vi "PROCESS_CTRL_VI.vi"(7 "simulazione":bool, 8 "error in (no error)":errorcluster, 10 "SINOTTICO NM":refnum<vi>, 11 "Queue Name":string) -> (0 "error out":errorcluster, 2 "Stopped":bool)   [LabVIEW 2016]
uses:
  TypeDef/Cluster MISURE.ctl
  TypeDef/MISURE NM.ctl
  TypeDef/Cluster misure ALL.ctl
  TypeDef/Cluster NI.ctl
  cDAQ_PLC Folder/controls/StatoAO_cdaq.ctl
  cDAQ_PLC Folder/controls/statoDO_Cdaq.ctl
  TypeDef/MISURE WT.ctl
  TypeDef/ClusterRes.ctl
  TypeDef/INTERFACCIA.ctl
  TypeDef/Lista AO sistema.ctl
  TypeDef/DOinterfaccia.ctl
  cDAQ_PLC Folder/ST1200_LIST_IO/STATO PLC 1.ctl
  cDAQ_PLC Folder/ST1200_LIST_IO/Uscite PLC 1.ctl
  cDAQ_PLC Folder/controls/statoAO_plc_1.ctl
  cDAQ_PLC Folder/ST1200_LIST_IO/StatoDO_PLC_1.ctl
  SINUS PENTA SANTERNO/controls/Parametri inverter letti.ctl
  TypeDef/SINOTTICO NM.ctl
  Globals.vi
panel:
  out "Setup pressione":dbl[](array[numeric])
  out "CTRL BV 3":cluster{"ON":bool, "OFF":bool}
  out "CTRL BV 2":cluster{"ON":bool, "OFF":bool}
  out "Stato Soglie":bool[](array[boolean])
  out "Pressione misurata":dbl
  out "Set Pressione":dbl
  out "Controllo Pressione":bool
  out "# in queue":i32
  out "STATO":string
  out "LOOP TIME (ms)":u32
  # "OK"
  # "BELOW RANGE"
  # "OVER RANGE"
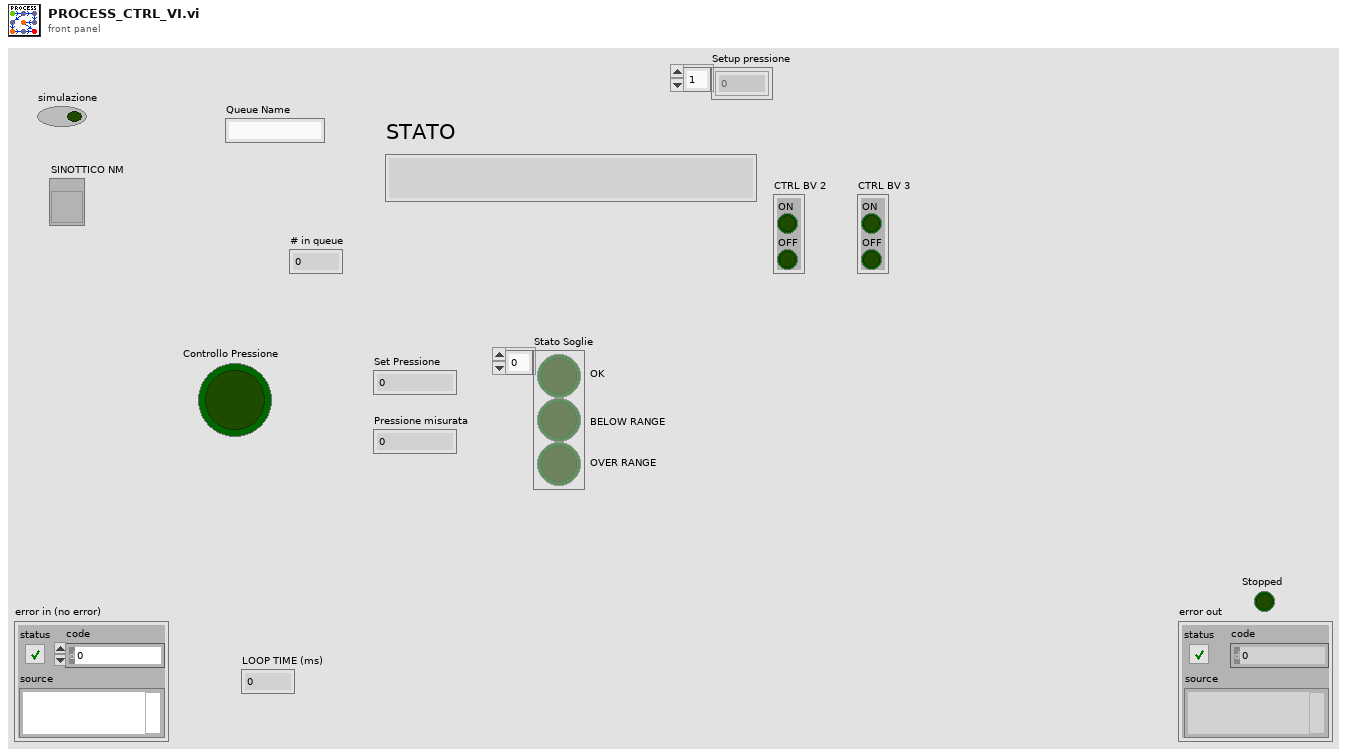
[diagram p1: front panel]
types:
  T1 = typedef "SINOTTICO NM.ctl" = cluster{"BooleanV 1":bool, "BooleanV 2":bool, "BooleanV 3":bool, "BooleanV 4":bool, "BooleanV 5":bool, "BooleanV 6":bool, "CTRL BV 2":cluster{"ON":bool, "OFF":bool}, "CTRL BV 3":cluster{"ON":bool, "OFF":bool}, "CTRL BV 4":cluster{"ON":bool, "OFF":bool}, "CTRL BV 5":cluster{"ON":bool, "OFF":bool}, "CTRL BV 6":cluster{"ON":bool, "OFF":bool}, "MTR 1":bool, "DN40%":dbl, "DN100%":dbl, "DN250%":dbl, "DN32":dbl, "DN100":dbl, "DN250":dbl, "MTR 2":bool, "BooleanV 7":bool, "BooleanV 8":bool, "DN25%":dbl, "DN250_c":dbl, "CTRL BV 7":cluster{"ON":bool, "OFF":bool}, "CTRL BV 8":cluster{"ON":bool, "OFF":bool}, "DN300%":dbl, "H 2 [bar]":dbl, "H 1 [bar]":dbl, "Rpm\nTorsiometro":dbl, "Coppia\nTorsiometro":dbl, "Sonda Velocità":dbl, "T 2 [°C]":dbl, "T 1 [°C]":dbl, "P [bar]":dbl, "Livello [m]":dbl, "MTR 3":bool, "SEL DN40":bool, "SEL DN100":bool, "SEL DN250":bool, "SEL DN300":bool, "SEL DN25":bool}
  T2 = typedef "Cluster MISURE.ctl" = cluster{"MISURE NM":T3, "MISURE ALL":T4}
  T3 = typedef "MISURE NM.ctl" = cluster{"Banco":string, "Anno":string, "Numero":string, "Ntabella":string, "Misura":string, "Tipo Prova":string, "ProgressivoAcq":string, "Descrizione":string, "Data_ora":string, "t. acq [h:m:s]":string, "t. acq [min]":string, "t. acq [s]":string, "n [rpm]":string, "f [Hz]":string, "U1[V]":string, "U2 [V]":string, "U3 [V]":string, "U123_media [V]":string, "I1[A]":string, "I2[A]":string, "I3[A]":string, "I123_media [A]*I":string, "I_123_sbil [%]":string, "Ulin[V]":string, "Uc [V]":string, "Uaux [V]":string, "Ilin[A]*I":string, "Imar[A]":string, "Iaux[A]":string, "Uarm[V]":string, "Uecc[V]":string, "Iarm[A]*I":string, "Iecc[A]":string, "pf":string, "P1 [W]":string, "P1 [kW]":string, "P1arm[W]":string, "P1ecc[W]":string, "Parm[kW]":string, "P1ecc[kW]":string, "Cond[uF]":string, "P1_linea_6fili[W]":string, "P1_linea_6fili[kW]":string, "eta_gr_6fili [%]":string, "eta_inverter_6fili [%]":string, "pf_linea_6fili":string, "U4 [V]":string, "U5 [V]":string, "U6 [V]":string, "U456_media [V]":string, "I4 [A]":string, "I5 [A]":string, "I6 [A]":string, "I456_media [A]":string, "C [Nm]*C":string, "Cric [Nm]":string, "Cric\\Cnom":string, "Iric[A]":string, "Iric\\Inom":string, "P2_mecc [W]":string, "P2_mecc [kW]":string, "eta motore [%]":string, "Scorr[%]":string, "Tamb[°C]":string, "R1[ohm]":string, "R2[ohm]":string, "R3[ohm]":string, "DT_R1[°C]":string, "DT_R2[°C]":string, "DT_R3[°C]":string, "R_marcia[ohm]":string, "R_aux[ohm]":string, "DT_marcia[°C]":string, "DT_aux[°C]":string, "R_Arm[ohm]":string, "R_Ecc[ohm]":string, "DT_Arm[°C]":string, "DT_Ecc[°C]":string, "TambFreddo[°C]":string, "R1_freddo[ohm]":string, "R2_freddo[ohm]":string, "R3_freddo[ohm]":string, "R_Marcia_freddo[ohm]":string, "R_Aux_freddo[ohm]":string, "R_Arm_freddo[ohm]":string, "R_Ecc_freddo[ohm]":string, "Tc1":string, "Tc2":string, "Tc3":string, "Tc4":string, "Tc5":string, "Tc6":string, "Tc7":string, "Tc8":string, "Vibr 1":string, "Vibr 2":string, "Vibr 3":string, "Scorta 1":string, "Scorta 2":string, "Scorta 3":string, "Scorta 4":string, "Scorta 5":string, "Scorta 6":string, "Scorta 7":string, "Scorta 8":string, "Scorta 9":string, "Scorta 10":string}
  T4 = typedef "Cluster misure ALL.ctl" = cluster{"Cluster READ NI":T5, "MISURE WT":T8, "Resistenze Resistomat":T9, "INTERFACCIA":T10, "FREDDO resistomat":cluster{"Res Ch1":dbl, "Res Ch2":dbl, "tAMB":dbl, "Res Ch3":dbl}, "STATO PLC":T15, "Res Ch2":dbl, "Res Ch2 2":dbl, "FREDDO res meter":cluster{"Res Ch1":dbl, "Res Ch2":dbl, "tAMB":dbl, "Res Ch3":dbl}, "Resistenze Res Meter":T9, "READ SINUS PENTA":T19}
  T5 = typedef "Cluster NI.ctl" = cluster{"AI (0-10V)":cluster{"AI 0":dbl, "AI 1":dbl, "AI 2":dbl, "AI 3":dbl, "AI 4":dbl, "AI 5":dbl, "AI 6":dbl, "AI 7":dbl, "AI 8":dbl, "AI 9":dbl, "AI 10":dbl, "AI 11":dbl, "AI 12":dbl, "AI 13":dbl, "AI 14":dbl, "AI 15":dbl, "AI 16":dbl, "AI 17":dbl, "AI 18":dbl, "AI 19":dbl, "AI 20":dbl, "AI 21":dbl, "AI 22":dbl, "AI 23":dbl, "AI 24":dbl, "AI 25":dbl, "AI 26":dbl, "AI 27":dbl, "AI 28":dbl, "AI 29":dbl, "AI 30":dbl, "AI 31":dbl}, "StatoAO_Cdaq[0-10V]":cluster{"AO 1":dbl, "AO 2":dbl, "AO 3":dbl, "AO 4":dbl}, "Contatori [rpm]":cluster{"RPM 1":dbl, "RPM 2":dbl}, "StatoAO_Cdaq [4-20mA]":T6, "StatoDO_Cdaq":T7, "DI":cluster{"Scorta 0":bool, "Scorta 1":bool, "Scorta 2":bool, "Scorta 3":bool, "Scorta 4":bool, "Scorta 5":bool, "Scorta 6":bool, "Scorta 7":bool, "Scorta 8":bool, "Scorta 9":bool, "Scorta 10":bool, "Scorta 11":bool, "Scorta 12":bool, "Scorta 13":bool, "Scorta 14":bool, "Scorta 15":bool, "Scorta 16":bool, "Scorta 17":bool, "Scorta 18":bool, "Scorta 19":bool, "Scorta 20":bool, "Scorta 21":bool, "Scorta 22":bool, "Scorta 23":bool, "Scorta 24":bool, "Scorta 25":bool, "Scorta 26":bool, "Scorta 27":bool, "Scorta 28":bool, "Scorta 29":bool, "Scorta 30":bool, "Scorta 31":bool}, "AI (4-20mA)":cluster{"AI 0":dbl, "AI 1":dbl, "AI 2":dbl, "AI 3":dbl, "AI 4":dbl, "AI 5":dbl, "AI 6":dbl, "AI 7":dbl, "AI 8":dbl, "AI 9":dbl, "AI 10":dbl, "AI 11":dbl, "AI 12":dbl, "AI 13":dbl, "AI 14":dbl, "AI 15":dbl}}
  T6 = typedef "StatoAO_cdaq.ctl" = cluster{"Cdaq_AO [0-10V] 0":dbl, "Cdaq_AO [0-10V] 1":dbl, "Cdaq_AO [0-10V] 2":dbl, "Cdaq_AO [0-10V] 3":dbl, "Cdaq_AO [4-20mA] 0":dbl, "Cdaq_AO [4-20mA] 1":dbl, "Cdaq_AO [4-20mA] 2":dbl, "Cdaq_AO [4-20mA] 3":dbl, "Cdaq_AO [4-20mA] 4":dbl, "Cdaq_AO [4-20mA] 5":dbl, "Cdaq_AO [4-20mA] 6":dbl, "Cdaq_AO [4-20mA] 7":dbl}
  T7 = typedef "statoDO_Cdaq.ctl" = cluster{"Scorta 0":bool, "Scorta 1":bool, "Scorta 2":bool, "Scorta 3":bool, "Scorta 4":bool, "Scorta 5":bool, "Scorta 6":bool, "Scorta 7":bool, "Scorta 8":bool, "Scorta 9":bool, "Scorta 10":bool, "Scorta 11":bool, "Scorta 12":bool, "Scorta 13":bool, "Scorta 14":bool, "Scorta 15":bool, "Scorta 16":bool, "Scorta 17":bool, "Scorta 18":bool, "Scorta 19":bool, "Scorta 20":bool, "Scorta 21":bool, "Scorta 22":bool, "Scorta 23":bool, "Scorta 24":bool, "Scorta 25":bool, "Scorta 26":bool, "Scorta 27":bool, "Scorta 28":bool, "Scorta 29":bool, "Scorta 30":bool, "Scorta 31":bool}
  T8 = typedef "MISURE WT.ctl" = cluster{"URMS 1":dbl, "IRMS 1":dbl, "P 1":dbl, "S 1":dbl, "Q 1":dbl, "LAMBDA 1":dbl, "PHI 1":dbl, "F U 1":dbl, "F I 1":dbl, "NONE 1":dbl, "URMS 2":dbl, "IRMS 2":dbl, "P 2":dbl, "S 2":dbl, "Q 2":dbl, "LAMBDA 2":dbl, "PHI 2":dbl, "F U 2":dbl, "F I 2":dbl, "NONE 2":dbl, "URMS 3":dbl, "IRMS 3":dbl, "P 3":dbl, "S 3":dbl, "Q 3":dbl, "LAMBDA 3":dbl, "PHI 3":dbl, "F U 3":dbl, "F I 3":dbl, "NONE 3":dbl, "URMS 4":dbl, "IRMS 4":dbl, "P 4":dbl, "S 4":dbl, "Q 4":dbl, "LAMBDA 4":dbl, "PHI 4":dbl, "F U 4":dbl, "F I 4":dbl, "NONE 4":dbl, "URMS 5":dbl, "IRMS 5":dbl, "P 5":dbl, "S 5":dbl, "Q 5":dbl, "LAMBDA 5":dbl, "PHI 5":dbl, "F U 5":dbl, "F I 5":dbl, "NONE 5":dbl, "URMS 6":dbl, "IRMS 6":dbl, "P 6":dbl, "S 6":dbl, "Q 6":dbl, "LAMBDA 6":dbl, "PHI 6":dbl, "F U 6":dbl, "F I 6":dbl, "NONE 6":dbl, "URMS SIGMA":dbl, "IRMS SIGMA":dbl, "P SIGMA":dbl, "S SIGMA":dbl, "Q SIGMA":dbl, "LAMBDA SIGMA":dbl, "PHI SIGMA":dbl, "F U SIGMA":dbl, "F I SIGMA":dbl, "NONE 7":dbl, "URMS SIGMB":dbl, "IRMS SIGMB":dbl, "P SIGMB":dbl, "S SIGMB":dbl, "Q SIGMB":dbl, "LAMBDA SIGMB":dbl, "PHI SIGMB":dbl, "F U SIGMB":dbl, "F I SIGMB":dbl, "NONE 8":dbl, "URMS SIGMC":dbl, "IRMS SIGMC":dbl, "P SIGMC":dbl, "S SIGMC":dbl, "Q SIGMC":dbl, "LAMBDA SIGMC":dbl, "PHI SIGMC":dbl, "F U SIGMC":dbl, "F I SIGMC":dbl, "NONE 9":dbl}
  T9 = typedef "ClusterRes.ctl" = cluster{"Res Ch1":dbl, "Res Ch2":dbl, "Res Ch3":dbl}
  T10 = typedef "INTERFACCIA.ctl" = cluster{"AI":cluster{"Portate":T11[], "Pressioni":T11[], "Coppie[Nm]":T11[], "Valvole prop %":T11[], "RPM":T11[], "Livelli":T11[], "Temperature":T11[], "Riferimenti %":T11[]}, "DI (logici)":cluster{"Start da pulsantiera":bool, "Stop da pulsantiera":bool, "Reset da pulsantiera":bool, "Sistema OK":bool, "Collaudo abilitato":bool, "Potenza trifase abilitata":bool, "Potenza monofase abilitata":bool, "Potenza DC abilitata":bool, "Potenza DC ECC abilitata":bool, "Start alimentazione AC":bool, "Start alimentazione DC":bool, "Start DC eccitazione":bool, "Teleruttore WT abilitato":bool, "Teleruttore Resistomat abilitato":bool, "Teleruttore corto fasi":bool, "Ramo 1 resistomat":bool, "Ramo 2 resistomat":bool, "Ramo 3 resistomat":bool, "Scelta linea elettrica 1":bool, "Scelta linea elettrica 2":bool, "Scelta linea elettrica 3":bool, "Scelta linea elettrica 4":bool, "Scelta linea elettrica 5":bool, "Rotore bloccato 1":bool, "Rotore bloccato 2":bool, "FRENO 1 abilitato":bool, "FRENO 1 run":bool, "FRENO 1 senso rotaz":bool, "FRENO 1 ctrl velocità":bool, "FRENO 2 abilitato":bool, "FRENO 2 run":bool, "FRENO 2 senso rotaz":bool, "FRENO 2 ctrl velocità":bool, "ALIM 1 abilitato":bool, "ALIM 1 run":bool, "ALIM 2 abilitato":bool, "ALIM 2 run":bool, "ALIM 3 abilitato":bool, "ALIM 3 run":bool, "FRENO 1 ctrl coppia":bool, "FRENO 2 ctrl coppia":bool, "FRENO 3 ctrl coppia":bool}, "AO non scalati":T13, "AO scalati":T13, "DO (logici)":T14, "DO aggiuntivi impianto":cluster{"Scorta 1":bool, "Scorta 2":bool, "Scorta 3":bool}}
  T11 = typedef "ClusterMisura_e_Unità_INPUT.ctl" = cluster{"Misura":dbl, "UM":T12, "Descrizione":string}
  T12 = typedef "UnitàMisura.ctl" = enum16{"V", "mA", "Bar", "RPM", "m3/s", "m3/min", "m3/h", "l/s", "l/min", "in3/min", "ft3/min", "gpm", "igpm", "igph", "%", "°C", "m", "Nm"}
  T13 = typedef "Lista AO sistema.ctl" = cluster{"FRENO1 rif vel":dbl, "FRENO1 rif Coppia":dbl, "FRENO2 rif vel":dbl, "FRENO2 rif Coppia":dbl, "ALIM1 rif V":dbl, "ALIM1 rif F":dbl, "ALIM2 rif V":dbl, "ALIM2 rif F":dbl, "ALIM3 rif V":dbl, "ALIM3 rif F":dbl}
  T14 = typedef "DOinterfaccia.ctl" = cluster{"Scelta banco 1":bool, "Scelta banco 2":bool, "Scelta banco 3":bool, "FRENO 1 abilita":bool, "FRENO 1 start":bool, "FRENO 1 senso rotaz":bool, "FRENO 1 ctrl velocità":bool, "FRENO 2 abilita":bool, "FRENO 2 start":bool, "FRENO 2 senso rotaz":bool, "FRENO 2 ctrl velocità":bool, "ALIM 1 abilita":bool, "ALIM 1 start":bool, "ALIM 2 abilita":bool, "ALIM 2 start":bool, "ALIM 3 abilita":bool, "ALIM 3 start":bool, "Abilita linea trifase":bool, "Abilita linea monofase":bool, "Abilita linea dc":bool, "Abilita linea dc eccit":bool, "Linea elettrica 1":bool, "Linea elettrica 2":bool, "Linea elettrica 3":bool, "Linea elettrica 4":bool, "Linea elettrica 5":bool, "Start potenza AC":bool, "Stop pontenza AC":bool, "Start potenza DC":bool, "Stop potenza DC":bool, "Start potenza eccitaz":bool, "Stop potenza eccitaz":bool, "Reset allarmi":bool, "watchdog":bool, "Scala torsiometro B1":bool, "Controllo torsiom B1":bool, "Scala torsiometro B2":bool, "Controllo torsiom B2":bool, "Teleruttore WT abilita":bool, "Teleruttore Resistomat abilita":bool, "Teleruttore corto fasi":bool, "Ramo 1 resistomat":bool, "Ramo 2 resistomat":bool, "Ramo 3 resistomat":bool, "Collaudo in corso":bool, "Allarme presente":bool, "Enable Res Meter":bool, "Bypass Res Meter":bool, "2nd canale Res Meter":bool, "Scala 200/2000 res meter":bool, "Taratura res meter":bool, "FRENO 1 ctrl coppia":bool, "FRENO 2 ctrl coppia":bool, "FRENO 3 ctrl coppia":bool, "Comando azionam in blocco":bool, "Comando azionam reset":bool, "Sensibilita freno 16 32nm":bool}
  T15 = typedef "STATO PLC 1.ctl" = cluster{"USCITE PLC":T16, "Stato DI_PLC":cluster{"Sistema OK":bool, "Sensore coppia di spunto":bool, "Variac man\\auto":bool, "Azionamento rmv>0":bool, "Linea 10A abilitata":bool, "Protezione azionamento 1":bool, "Linea 63A selezionata":bool, "Motore alimentato":bool, "Scelta monofase":bool, "Scelta trifase":bool, "Scorta 5":bool, "Scorta 6":bool, "Scorta 7":bool, "Scorta 8":bool, "Scorta 9":bool, "Scorta 10":bool}, "AI plc":cluster{"Allarmi 1":dbl, "Allarmi 2":dbl, "Stato condensatori":dbl}}
  T16 = typedef "Uscite PLC 1.ctl" = cluster{"AO (real) 2":cluster{"SCORTA 1":dbl, "SCORTA 2":dbl, "SCORTA 3":dbl, "SCORTA 4":dbl, "SCORTA 5":dbl, "SCORTA 6":dbl, "SCORTA 7":dbl, "SCORTA 8":dbl}, "statoAO_PLC out":T17, "DO (bit)":T18}
  T17 = typedef "statoAO_plc_1.ctl" = cluster{"Condensatori":dbl, "Scorta 1":dbl, "Scorta 2":dbl, "Scorta 3":dbl}
  T18 = typedef "StatoDO_PLC_1.ctl" = cluster{"Selezione banco 1":bool, "Selezione trifase\\monofase":bool, "Abilita linea 63A":bool, "Sensibilità 16/32":bool, "Scala 200/2000 res meter":bool, "Taratura res meter":bool, "Start azionamento":bool, "Comando start azion in corrente":bool, "Comando start azion in giri":bool, "Comando azion in blocco":bool, "Comando azion reset":bool, "Senso rotazione":bool, "Rif corrente giri costanti":bool, "Allarme":bool, "Abilita TA 60/1A":bool, "Abilita TA 10/1 A":bool, "Abilita linea 10A":bool, "Watchdog":bool, "START MOTORE":bool, "Scorta 2":bool, "Scorta 3":bool, "Scorta 4":bool, "Scorta 5":bool, "Scorta 6":bool}
  T19 = typedef "Parametri inverter letti.ctl" = cluster{"Menù Misure motore (M000-M030)":cluster{"Rif vel a regime (int)":u16, "Rif vel a regime (dec)":u16, "Rif vel dopo rampe (int)":u16, "Rif vel dopo rampe (dec)":u16, "RPM motore (int)":u16, "RPM motore (dec)":u16, "FREQout inverter":u16, "Rif coppia a regime(Nm)":u16, "Richiesta di coppia (Nm)":u16, "Coppia generata dal motore(Nm)":u16, "Rif coppia a regime(%)":u16, "Richiesta di coppia (%)":u16, "Coppia generata dal motore(%)":u16, "Coppia max richiesta prima delle rampe(Nm)":u16, "Coppia max richiesta dopo le rampe(Nm)":u16, "Limite di velocità prima delle rampe":u16, "Limite di velocità dopo le rampe":u16, "Coppia max richiesta prima delle rampe(%)":u16, "Coppia max richiesta dopo le rampe(%)":u16, "Rif di flusso":u16, "Corrente di uscita":u16, "Capacità termica del motore":u16, "Tensione di uscita":u16, "Potenza di uscita":u16, "Energia consumata (LSword)":u16, "Energia consumata (MSword)":u16, "Tensione bus DC":u16, "Tensione di rete":u16}, "Menù regolatore PID (M018-M024)":cluster{"Rif PID a regime(%)":u16, "Rif pid dopo rampe(%)":u16, "Retroazione del pid(%)":u16, "Errore del pid(%)":u16, "uscita del pid(%)":u16, "Rif del pid dopo le rampe":u16, "Retroazione del pid":u16}, "Menù ingressi digitali (M031-M036)":cluster{"Ingressi digitali ritardati":u16, "Ingressi digitali istantanei":u16, "Moresettiera comando loc":u16, "Morsett comando da seriale":u16, "Morsett comando bus di campo":u16, "Ing dig ausiliari da morsettiera":u16, "Ing dig ausiliari da seriale":u16}, "Menù riferimenti (M037-M051)":cluster{"Rif analog est REF":u16, "Rif analog est AIN1":u16, "Rif analog est AIN2":u16, "Rif analog est XAIN4":u16, "Rif analog est XAIN5":u16, "Rif velocità da seriale(int)":u16, "Rif velocità bus di campo(int)":u16, "Rif coppia da seriale":u16, "Rif coppia bus di campo":u16, "Rif del PID da seriale":u16, "Rif del PID da bus di campo":u16, "Retroazione del PID da seriale":u16, "Retroazione del PIDda bus di campo":u16, "Rif da encoder":u16, "Rif in frequenza":u16, "Rif velocità da seriale(dec)":u16, "Rif velocità bus di campo(dec)":u16}, "Menù rampe (P009-P033)":cluster{"Tempo di dec rampa di vel 1":u16, "Tempo di acc rampa di vel 2":u16, "Tempo di dec rampa di vel 2":u16, "Tempo di acc rampa di vel 1":u16, "Unità di mis tempi rampe vel 1/2":u16, "Tempo di acc rampa di vel 3":u16, "Tempo di dec rampa di vel 3":u16, "Tempo di acc rampa di vel 4":u16, "Tempo di dec rampa di vel 4":u16, "Unità di mis tempi rampe vel 3/4":u16, "Selettore arrottondam rampe":u16, "Tempo di arrotond iniz rampa acc":u16, "Tempo di arrotond finale rampa acc":u16, "Tempo di arrotond iniz rampa dec":u16, "Tempo di rampa di salita rif coppia":u16, "Tempo di rampa di discesa rif coppia":u16, "Unità di misura rampa coppia":u16, "Tempo rampa acc marcia jog":u16, "Tempo rampa dec marcia jog":u16, "Reset acc ai cambi pendenza":u16, "rampa di acc in fire mode":u16, "rampa di dec in fire mode":u16, "Tempo di arrotond finale rampa dec":u16}, "Menù controllo motore(C008-C128)":cluster{"Numero motori configurati":u16, "Tipo algoritmo di controllo Mot1":u16, "Tipo rif Mot1":u16, "Tensione nominale rete":u16, "Retroaz di vel da encoder Mot1":u16, "Tipo curva V/f Mot1":u16, "Rotazione delle fasi Mot1":u16, "Freq nominale del motore Mot1":u16, "RPM nominali del motore Mot1":u16, "Potenza nominale del motore Mot1":u16, "Corrente nominale del motore Mot1":u16, "Tensione nominale del motore mot1":u16, "Potenza a vuoto del motore Mot1":u16, "Corrente a vuoto del motore Mot1":u16, "Resistenza statorica del motore Mot1":u16, "Induttanza di dispersione Mot1":u16}, "Menù configurazione PID":cluster{"Selezione riferimento n.1":u16, "Selezione retroazione n.1":u16, "Modalità di fuzionamento PID":u16, "Termine derivativo calcolato su err o mis":u16, "Proporz moltiplica deriv e integrale":u16, "Azione del PID":u16}, "ID":dbl, "Menù uscite digitali":cluster{"MDO4 Inverter pronto":u16}, "Fcarrier":cluster{"Fcarrier Min (Hz)":u16, "Fcarrier Max (Hz)":u16}, "stato inverter M089":dbl, "Riferimenti":cluster{"Rif tensione":u16, "Rif velocità":u16}}
  T20 = cluster{"CLUSTER PROCESSI":cluster{"Controllo\nPressione":bool, "Pressione\nassoluta [bar]":dbl}, "Cluster MISURE":T2}
  T21 = enum32{"Invalid", "Standard", "Closed", "Hidden", "Minimized", "Maximized"}
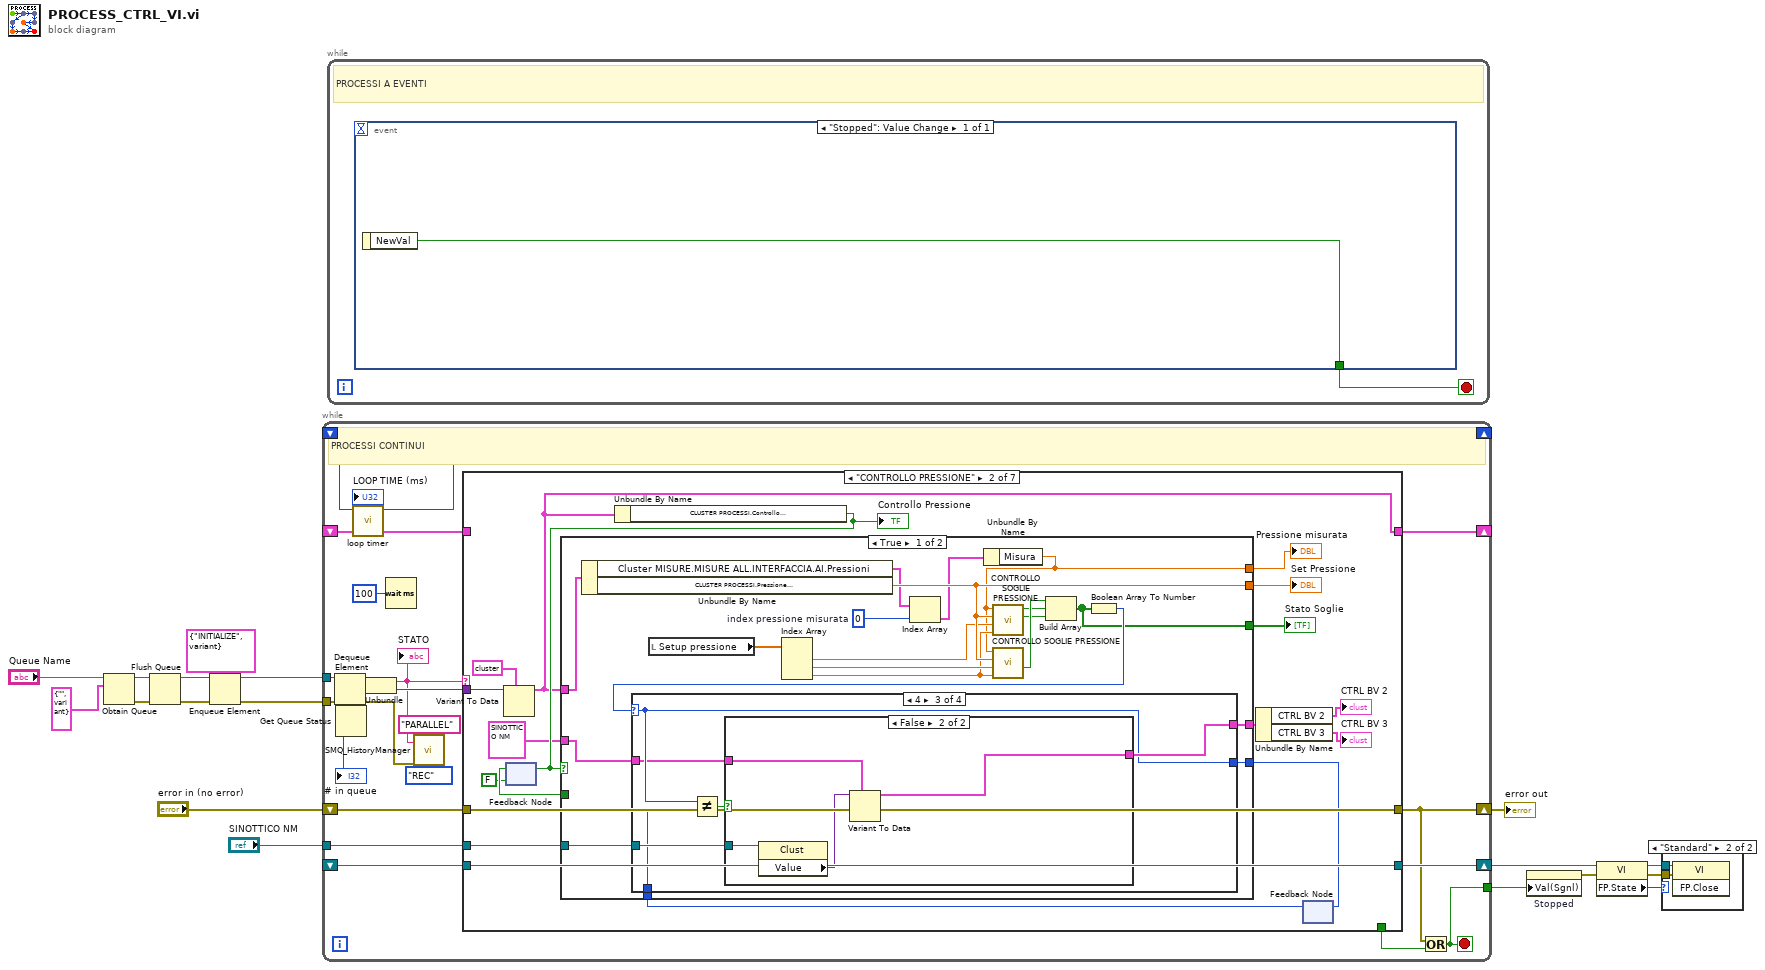
[diagram p0: block diagram]
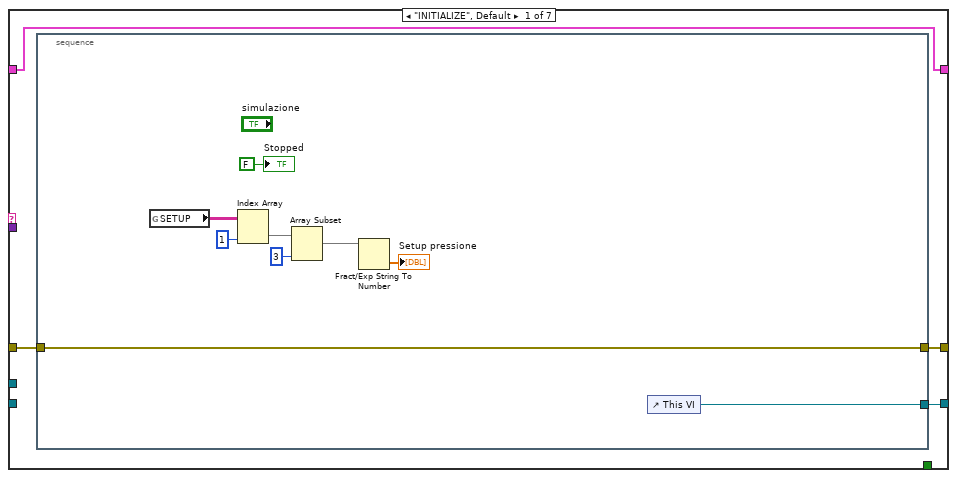
[diagram p3: hidden frame]
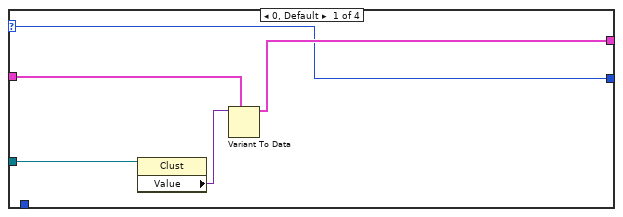
[diagram p4: hidden frame]
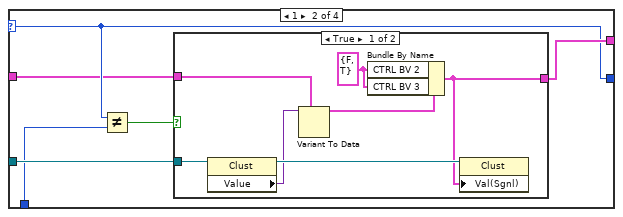
[diagram p5: hidden frame]
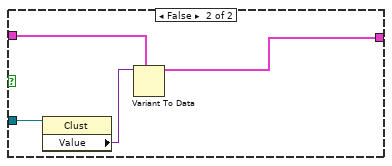
[diagram p6: hidden frame]
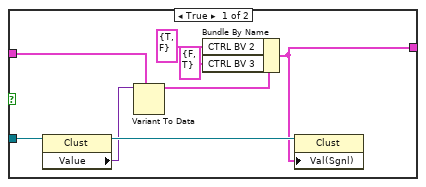
[diagram p7: hidden frame]
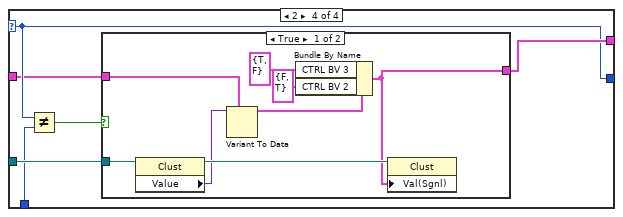
[diagram p8: hidden frame]
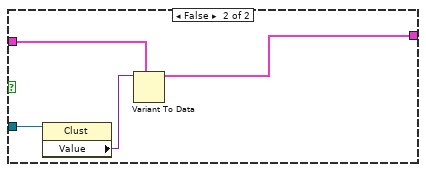
[diagram p9: hidden frame]
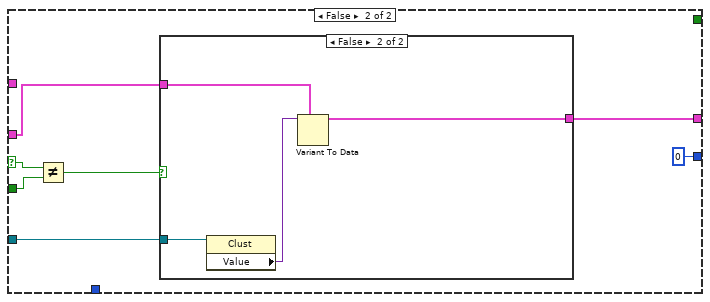
[diagram p10: hidden frame]
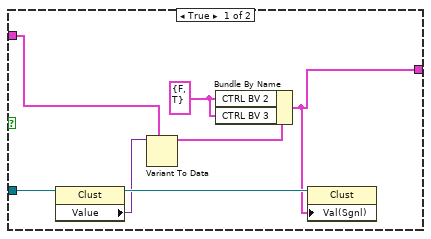
[diagram p11: hidden frame]
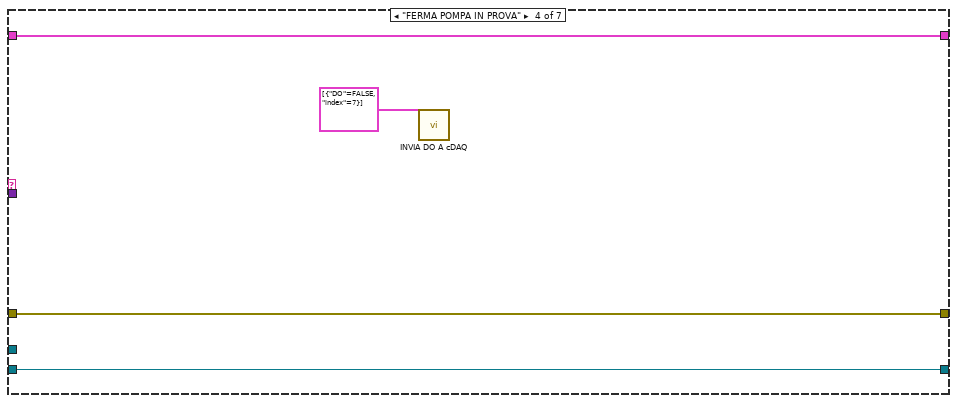
[diagram p13: hidden frame]
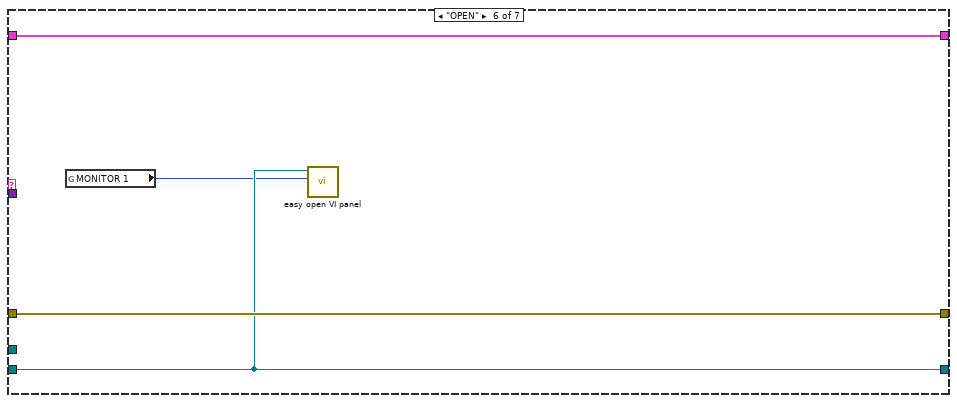
[diagram p15: hidden frame]
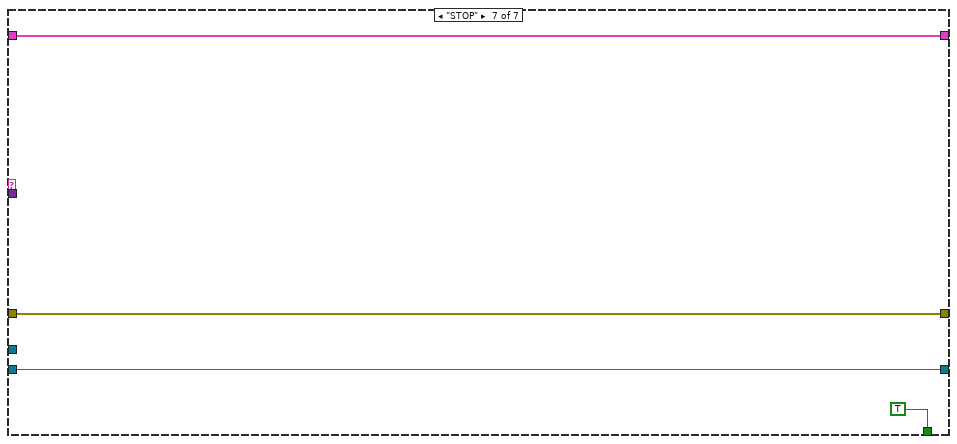
[diagram p16: hidden frame]
diagram:
  n1 = Obtain Queue(name (unnamed)="Queue Name", element data type=cluster{"String":string, "variant":variant} {"String"="", "variant"=variant} ("element")) -> (queue out=w6:refnum<queue>, error out=w5:errorcluster)  [unwired: 3 in, 1 out]
  n2 = Flush Queue(queue=w6, error in (no error)=w5) -> (queue out=w3:refnum<queue>, error out=w2:errorcluster)  [unwired: 1 out]
  n3 = Enqueue Element(queue=w3, element=cluster{"String":string, "variant":variant} {"String"="INITIALIZE", "variant"=variant}, error in (no error)=w2) -> (queue out=w8:refnum<queue>, error out=w7:errorcluster)  [unwired: 1 in, 1 out]
  n4 = while {
    shift-right: [w41] -> _
    shift-left: _ -> [w40]
    shift-right: [w38] -> w11
    shift-left: _ -> [w37]
    shift-right: [w34] -> w14
    shift-left: "error in (no error)" -> [w36]
    tunnel: w8 -> [w32]
    tunnel: w7 -> [w33]
    tunnel: [w29] -> w15
    tunnel: "SINOTTICO NM" -> [w21]
    shift-right: [w20] -> _
    shift-left: _ -> [w19]
    stop <- w29 stop-if-true
    # "PROCESSI CONTINUI"
    n5 = Dequeue Element(queue=w32, error in (no error)=w33) -> (queue out=w24:refnum<queue>, element=w31:cluster{"String":string, "variant":variant}, error out=w26:errorcluster)  [unwired: 1 in, 1 out]
    n6 = Get Queue Status(queue=w24) -> (# elements in queue=→"# in queue":i32)  [unwired: 2 in, 7 out]
    n7 = call <userlib>:"loop timer.vi"("millisecond timer IN"=w40) -> ("millisecond timer OUT"=w41:u32, "LOOP TIME (ms)"=→"LOOP TIME (ms)":u32)  [unwired: 9 in]
    n8 = Unbundle(w31) -> ("String"=w27:string, "variant"=w30:variant)
    "STATO" <- w27
    n9 = Wait (ms)(milliseconds to wait=u32 100) -> ()  [unwired: 1 out]
    n10 = call <userlib>:"SMQ_HistoryManager.vi"("Caller VI"="PARALLEL", "State"=w27, "error in (no error)"=w26, "Function"=enum16{"INITIALIZE", "REC", "STOP"}."REC") -> ()  [unwired: 14 in, 2 out]
    n11 = case shown="\"CONTROLLO PRESSIONE\"" w27 {
      tunnel: [_ _ _ _ _ _ TRUE] -> w35
      tunnel: [w45 w72 w171 w175 w178 w181 w185] -> w38
      tunnel: w37 -> [_ w72 w171 w175 w178 w181 w185]
      tunnel: w36 -> [w44 w63 w170 w174 w177 w182 w184]
      tunnel: [w43 w63 w170 w174 w177 w182 w184] -> w34
      tunnel: w30 -> [_ w71 _ _ _ _ _]
      tunnel: w21 -> [_ w70 _ _ _ _ _]
      tunnel: [w42 w55 w169 w172 w176 w179 w183] -> w20
      tunnel: w19 -> [w42 _ w169 w172 w176 w179 w183]
      frame "INITIALIZE", Default {
        n12 = stacked-sequence {
          tunnel: [w54] -> w45
          tunnel: w44 -> [w52]
          tunnel: [w52] -> w43
          frame #0 {
            n13 = global read "Globals.vi" "SETUP"() -> (w51:string[][])
            n14 = Index Array(array=w51, index (col)=1 ("disabled index (col)")) -> (element=w48:string[])  [unwired: 1 in]
            n15 = Array Subset(array=w48, length=3) -> (w46:string[])  [unwired: 1 in]
            n16 = Fract/Exp String To Number(string=w46) -> (number=→"Setup pressione":dbl[])  [unwired: 3 in, 1 out]
            n17 = control-ref of="This VI"() -> (w54:refnum<vi>)
            "Stopped" <- FALSE ("Stop")
          }
        }
      }
      frame "CONTROLLO PRESSIONE" {
        n18 = Variant To Data(type=T20 {"CLUSTER PROCESSI"={"Controllo\nPressione"=FALSE, "Pressione\nassoluta [bar]"=0.0}, "Cluster MISURE"={"MISURE NM"={"Banco"="", "Anno"="", "Numero"="", "Ntabella"="", "Misura"="", "Tipo Prova"="", "ProgressivoAcq"="", "Descrizione"="", "Data_ora"="", "t. acq [h:m:s]"="", "t. acq [min]"="", "t. acq [s]"="", "n [rpm]"="", "f [Hz]"="", "U1[V]"="", "U2 [V]"="", "U3 [V]"="", "U123_media [V]"="", "I1[A]"="", "I2[A]"="", "I3[A]"="", "I123_media [A]*I"="", "I_123_sbil [%]"="", "Ulin[V]"="", "Uc [V]"="", "Uaux [V]"="", "Ilin[A]*I"="", "Imar[A]"="", "Iaux[A]"="", "Uarm[V]"="", "Uecc[V]"="", "Iarm[A]*I"="", "Iecc[A]"="", "pf"="", "P1 [W]"="", "P1 [kW]"="", "P1arm[W]"="", "P1ecc[W]"="", "Parm[kW]"="", "P1ecc[kW]"="", "Cond[uF]"="", "P1_linea_6fili[W]"="", "P1_linea_6fili[kW]"="", "eta_gr_6fili [%]"="", "eta_inverter_6fili [%]"="", "pf_linea_6fili"="", "U4 [V]"="", "U5 [V]"="", "U6 [V]"="", "U456_media [V]"="", "I4 [A]"="", "I5 [A]"="", "I6 [A]"="", "I456_media [A]"="", "C [Nm]*C"="", "Cric [Nm]"="", "Cric\\Cnom"="", "Iric[A]"="", "Iric\\Inom"="", "P2_mecc [W]"="", "P2_mecc [kW]"="", "eta motore [%]"="", "Scorr[%]"="", "Tamb[°C]"="", "R1[ohm]"="", "R2[ohm]"="", "R3[ohm]"="", "DT_R1[°C]"="", "DT_R2[°C]"="", "DT_R3[°C]"="", "R_marcia[ohm]"="", "R_aux[ohm]"="", "DT_marcia[°C]"="", "DT_aux[°C]"="", "R_Arm[ohm]"="", "R_Ecc[ohm]"="", "DT_Arm[°C]"="", "DT_Ecc[°C]"="", "TambFreddo[°C]"="", "R1_freddo[ohm]"="", "R2_freddo[ohm]"="", "R3_freddo[ohm]"="", "R_Marcia_freddo[ohm]"="", "R_Aux_freddo[ohm]"="", "R_Arm_freddo[ohm]"="", "R_Ecc_freddo[ohm]"="", "Tc1"="", "Tc2"="", "Tc3"="", "Tc4"="", "Tc5"="", "Tc6"="", "Tc7"="", "Tc8"="", "Vibr 1"="", "Vibr 2"="", "Vibr 3"="", "Scorta 1"="", "Scorta 2"="", "Scorta 3"="", "Scorta 4"="", "Scorta 5"="", "Scorta 6"="", "Scorta 7"="", "Scorta 8"="", "Scorta 9"="", "Scorta 10"=""}, "MISURE ALL"={"Cluster READ NI"={"AI (0-10V)"={"AI 0"=0.0, "AI 1"=0.0, "AI 2"=0.0, "AI 3"=0.0, "AI 4"=0.0, "AI 5"=0.0, "AI 6"=0.0, "AI 7"=0.0, "AI 8"=0.0, "AI 9"=0.0, "AI 10"=0.0, "AI 11"=0.0, "AI 12"=0.0, "AI 13"=0.0, "AI 14"=0.0, "AI 15"=0.0, "AI 16"=0.0, "AI 17"=0.0, "AI 18"=0.0, "AI 19"=0.0, "AI 20"=0.0, "AI 21"=0.0, "AI 22"=0.0, "AI 23"=0.0, "AI 24"=0.0, "AI 25"=0.0, "AI 26"=0.0, "AI 27"=0.0, "AI 28"=0.0, "AI 29"=0.0, "AI 30"=0.0, "AI 31"=0.0}, "StatoAO_Cdaq[0-10V]"={"AO 1"=0.0, "AO 2"=0.0, "AO 3"=0.0, "AO 4"=0.0}, "Contatori [rpm]"={"RPM 1"=0.0, "RPM 2"=0.0}, "StatoAO_Cdaq [4-20mA]"={"Cdaq_AO [0-10V] 0"=0.0, "Cdaq_AO [0-10V] 1"=0.0, "Cdaq_AO [0-10V] 2"=0.0, "Cdaq_AO [0-10V] 3"=0.0, "Cdaq_AO [4-20mA] 0"=0.0, "Cdaq_AO [4-20mA] 1"=0.0, "Cdaq_AO [4-20mA] 2"=0.0, "Cdaq_AO [4-20mA] 3"=0.0, "Cdaq_AO [4-20mA] 4"=0.0, "Cdaq_AO [4-20mA] 5"=0.0, "Cdaq_AO [4-20mA] 6"=0.0, "Cdaq_AO [4-20mA] 7"=0.0}, "StatoDO_Cdaq"={"Scorta 0"=FALSE, "Scorta 1"=FALSE, "Scorta 2"=FALSE, "Scorta 3"=FALSE, "Scorta 4"=FALSE, "Scorta 5"=FALSE, "Scorta 6"=FALSE, "Scorta 7"=FALSE, "Scorta 8"=FALSE, "Scorta 9"=FALSE, "Scorta 10"=FALSE, "Scorta 11"=FALSE, "Scorta 12"=FALSE, "Scorta 13"=FALSE, "Scorta 14"=FALSE, "Scorta 15"=FALSE, "Scorta 16"=FALSE, "Scorta 17"=FALSE, "Scorta 18"=FALSE, "Scorta 19"=FALSE, "Scorta 20"=FALSE, "Scorta 21"=FALSE, "Scorta 22"=FALSE, "Scorta 23"=FALSE, "Scorta 24"=FALSE, "Scorta 25"=FALSE, "Scorta 26"=FALSE, "Scorta 27"=FALSE, "Scorta 28"=FALSE, "Scorta 29"=FALSE, "Scorta 30"=FALSE, "Scorta 31"=FALSE}, "DI"={"Scorta 0"=FALSE, "Scorta 1"=FALSE, "Scorta 2"=FALSE, "Scorta 3"=FALSE, "Scorta 4"=FALSE, "Scorta 5"=FALSE, "Scorta 6"=FALSE, "Scorta 7"=FALSE, "Scorta 8"=FALSE, "Scorta 9"=FALSE, "Scorta 10"=FALSE, "Scorta 11"=FALSE, "Scorta 12"=FALSE, "Scorta 13"=FALSE, "Scorta 14"=FALSE, "Scorta 15"=FALSE, "Scorta 16"=FALSE, "Scorta 17"=FALSE, "Scorta 18"=FALSE, "Scorta 19"=FALSE, "Scorta 20"=FALSE, "Scorta 21"=FALSE, "Scorta 22"=FALSE, "Scorta 23"=FALSE, "Scorta 24"=FALSE, "Scorta 25"=FALSE, "Scorta 26"=FALSE, "Scorta 27"=FALSE, "Scorta 28"=FALSE, "Scorta 29"=FALSE, "Scorta 30"=FALSE, "Scorta 31"=FALSE}, "AI (4-20mA)"={"AI 0"=0.0, "AI 1"=0.0, "AI 2"=0.0, "AI 3"=0.0, "AI 4"=0.0, "AI 5"=0.0, "AI 6"=0.0, "AI 7"=0.0, "AI 8"=0.0, "AI 9"=0.0, "AI 10"=0.0, "AI 11"=0.0, "AI 12"=0.0, "AI 13"=0.0, "AI 14"=0.0, "AI 15"=0.0}}, "MISURE WT"={"URMS 1"=0.0, "IRMS 1"=0.0, "P 1"=0.0, "S 1"=0.0, "Q 1"=0.0, "LAMBDA 1"=0.0, "PHI 1"=0.0, "F U 1"=0.0, "F I 1"=0.0, "NONE 1"=0.0, "URMS 2"=0.0, "IRMS 2"=0.0, "P 2"=0.0, "S 2"=0.0, "Q 2"=0.0, "LAMBDA 2"=0.0, "PHI 2"=0.0, "F U 2"=0.0, "F I 2"=0.0, "NONE 2"=0.0, "URMS 3"=0.0, "IRMS 3"=0.0, "P 3"=0.0, "S 3"=0.0, "Q 3"=0.0, "LAMBDA 3"=0.0, "PHI 3"=0.0, "F U 3"=0.0, "F I 3"=0.0, "NONE 3"=0.0, "URMS 4"=0.0, "IRMS 4"=0.0, "P 4"=0.0, "S 4"=0.0, "Q 4"=0.0, "LAMBDA 4"=0.0, "PHI 4"=0.0, "F U 4"=0.0, "F I 4"=0.0, "NONE 4"=0.0, "URMS 5"=0.0, "IRMS 5"=0.0, "P 5"=0.0, "S 5"=0.0, "Q 5"=0.0, "LAMBDA 5"=0.0, "PHI 5"=0.0, "F U 5"=0.0, "F I 5"=0.0, "NONE 5"=0.0, "URMS 6"=0.0, "IRMS 6"=0.0, "P 6"=0.0, "S 6"=0.0, "Q 6"=0.0, "LAMBDA 6"=0.0, "PHI 6"=0.0, "F U 6"=0.0, "F I 6"=0.0, "NONE 6"=0.0, "URMS SIGMA"=0.0, "IRMS SIGMA"=0.0, "P SIGMA"=0.0, "S SIGMA"=0.0, "Q SIGMA"=0.0, "LAMBDA SIGMA"=0.0, "PHI SIGMA"=0.0, "F U SIGMA"=0.0, "F I SIGMA"=0.0, "NONE 7"=0.0, "URMS SIGMB"=0.0, "IRMS SIGMB"=0.0, "P SIGMB"=0.0, "S SIGMB"=0.0, "Q SIGMB"=0.0, "LAMBDA SIGMB"=0.0, "PHI SIGMB"=0.0, "F U SIGMB"=0.0, "F I SIGMB"=0.0, "NONE 8"=0.0, "URMS SIGMC"=0.0, "IRMS SIGMC"=0.0, "P SIGMC"=0.0, "S SIGMC"=0.0, "Q SIGMC"=0.0, "LAMBDA SIGMC"=0.0, "PHI SIGMC"=0.0, "F U SIGMC"=0.0, "F I SIGMC"=0.0, "NONE 9"=0.0}, "Resistenze Resistomat"={"Res Ch1"=0.0, "Res Ch2"=0.0, "Res Ch3"=0.0}, "INTERFACCIA"={"AI"={"Portate"=[], "Pressioni"=[], "Coppie[Nm]"=[], "Valvole prop %"=[], "RPM"=[], "Livelli"=[], "Temperature"=[], "Riferimenti %"=[]}, "DI (logici)"={"Start da pulsantiera"=FALSE, "Stop da pulsantiera"=FALSE, "Reset da pulsantiera"=FALSE, "Sistema OK"=FALSE, "Collaudo abilitato"=FALSE, "Potenza trifase abilitata"=FALSE, "Potenza monofase abilitata"=FALSE, "Potenza DC abilitata"=FALSE, "Potenza DC ECC abilitata"=FALSE, "Start alimentazione AC"=FALSE, "Start alimentazione DC"=FALSE, "Start DC eccitazione"=FALSE, "Teleruttore WT abilitato"=FALSE, "Teleruttore Resistomat abilitato"=FALSE, "Teleruttore corto fasi"=FALSE, "Ramo 1 resistomat"=FALSE, "Ramo 2 resistomat"=FALSE, "Ramo 3 resistomat"=FALSE, "Scelta linea elettrica 1"=FALSE, "Scelta linea elettrica 2"=FALSE, "Scelta linea elettrica 3"=FALSE, "Scelta linea elettrica 4"=FALSE, "Scelta linea elettrica 5"=FALSE, "Rotore bloccato 1"=FALSE, "Rotore bloccato 2"=FALSE, "FRENO 1 abilitato"=FALSE, "FRENO 1 run"=FALSE, "FRENO 1 senso rotaz"=FALSE, "FRENO 1 ctrl velocità"=FALSE, "FRENO 2 abilitato"=FALSE, "FRENO 2 run"=FALSE, "FRENO 2 senso rotaz"=FALSE, "FRENO 2 ctrl velocità"=FALSE, "ALIM 1 abilitato"=FALSE, "ALIM 1 run"=FALSE, "ALIM 2 abilitato"=FALSE, "ALIM 2 run"=FALSE, "ALIM 3 abilitato"=FALSE, "ALIM 3 run"=FALSE, "FRENO 1 ctrl coppia"=FALSE, "FRENO 2 ctrl coppia"=FALSE, "FRENO 3 ctrl coppia"=FALSE}, "AO non scalati"={"FRENO1 rif vel"=0.0, "FRENO1 rif Coppia"=0.0, "FRENO2 rif vel"=0.0, "FRENO2 rif Coppia"=0.0, "ALIM1 rif V"=0.0, "ALIM1 rif F"=0.0, "ALIM2 rif V"=0.0, "ALIM2 rif F"=0.0, "ALIM3 rif V"=0.0, "ALIM3 rif F"=0.0}, "AO scalati"={"FRENO1 rif vel"=0.0, "FRENO1 rif Coppia"=0.0, "FRENO2 rif vel"=0.0, "FRENO2 rif Coppia"=0.0, "ALIM1 rif V"=0.0, "ALIM1 rif F"=0.0, "ALIM2 rif V"=0.0, "ALIM2 rif F"=0.0, "ALIM3 rif V"=0.0, "ALIM3 rif F"=0.0}, "DO (logici)"={"Scelta banco 1"=FALSE, "Scelta banco 2"=FALSE, "Scelta banco 3"=FALSE, "FRENO 1 abilita"=FALSE, "FRENO 1 start"=FALSE, "FRENO 1 senso rotaz"=FALSE, "FRENO 1 ctrl velocità"=FALSE, "FRENO 2 abilita"=FALSE, "FRENO 2 start"=FALSE, "FRENO 2 senso rotaz"=FALSE, "FRENO 2 ctrl velocità"=FALSE, "ALIM 1 abilita"=FALSE, "ALIM 1 start"=FALSE, "ALIM 2 abilita"=FALSE, "ALIM 2 start"=FALSE, "ALIM 3 abilita"=FALSE, "ALIM 3 start"=FALSE, "Abilita linea trifase"=FALSE, "Abilita linea monofase"=FALSE, "Abilita linea dc"=FALSE, "Abilita linea dc eccit"=FALSE, "Linea elettrica 1"=FALSE, "Linea elettrica 2"=FALSE, "Linea elettrica 3"=FALSE, "Linea elettrica 4"=FALSE, "Linea elettrica 5"=FALSE, "Start potenza AC"=FALSE, "Stop pontenza AC"=FALSE, "Start potenza DC"=FALSE, "Stop potenza DC"=FALSE, "Start potenza eccitaz"=FALSE, "Stop potenza eccitaz"=FALSE, "Reset allarmi"=FALSE, "watchdog"=FALSE, "Scala torsiometro B1"=FALSE, "Controllo torsiom B1"=FALSE, "Scala torsiometro B2"=FALSE, "Controllo torsiom B2"=FALSE, "Teleruttore WT abilita"=FALSE, "Teleruttore Resistomat abilita"=FALSE, "Teleruttore corto fasi"=FALSE, "Ramo 1 resistomat"=FALSE, "Ramo 2 resistomat"=FALSE, "Ramo 3 resistomat"=FALSE, "Collaudo in corso"=FALSE, "Allarme presente"=FALSE, "Enable Res Meter"=FALSE, "Bypass Res Meter"=FALSE, "2nd canale Res Meter"=FALSE, "Scala 200/2000 res meter"=FALSE, "Taratura res meter"=FALSE, "FRENO 1 ctrl coppia"=FALSE, "FRENO 2 ctrl coppia"=FALSE, "FRENO 3 ctrl coppia"=FALSE, "Comando azionam in blocco"=FALSE, "Comando azionam reset"=FALSE, "Sensibilita freno 16 32nm"=FALSE}, "DO aggiuntivi impianto"={"Scorta 1"=FALSE, "Scorta 2"=FALSE, "Scorta 3"=FALSE}}, "FREDDO resistomat"={"Res Ch1"=0.0, "Res Ch2"=0.0, "tAMB"=0.0, "Res Ch3"=0.0}, "STATO PLC"={"USCITE PLC"={"AO (real) 2"={"SCORTA 1"=0.0, "SCORTA 2"=0.0, "SCORTA 3"=0.0, "SCORTA 4"=0.0, "SCORTA 5"=0.0, "SCORTA 6"=0.0, "SCORTA 7"=0.0, "SCORTA 8"=0.0}, "statoAO_PLC out"={"Condensatori"=nan, "Scorta 1"=nan, "Scorta 2"=0.0, "Scorta 3"=0.0}, "DO (bit)"={"Selezione banco 1"=FALSE, "Selezione trifase\\monofase"=FALSE, "Abilita linea 63A"=FALSE, "Sensibilità 16/32"=FALSE, "Scala 200/2000 res meter"=FALSE, "Taratura res meter"=FALSE, "Start azionamento"=FALSE, "Comando start azion in corrente"=FALSE, "Comando start azion in giri"=FALSE, "Comando azion in blocco"=FALSE, "Comando azion reset"=FALSE, "Senso rotazione"=FALSE, "Rif corrente giri costanti"=FALSE, "Allarme"=FALSE, "Abilita TA 60/1A"=FALSE, "Abilita TA 10/1 A"=FALSE, "Abilita linea 10A"=FALSE, "Watchdog"=FALSE, "START MOTORE"=FALSE, "Scorta 2"=FALSE, "Scorta 3"=FALSE, "Scorta 4"=FALSE, "Scorta 5"=FALSE, "Scorta 6"=FALSE}}, "Stato DI_PLC"={"Sistema OK"=FALSE, "Sensore coppia di spunto"=FALSE, "Variac man\\auto"=FALSE, "Azionamento rmv>0"=FALSE, "Linea 10A abilitata"=FALSE, "Protezione azionamento 1"=FALSE, "Linea 63A selezionata"=FALSE, "Motore alimentato"=FALSE, "Scelta monofase"=FALSE, "Scelta trifase"=FALSE, "Scorta 5"=FALSE, "Scorta 6"=FALSE, "Scorta 7"=FALSE, "Scorta 8"=FALSE, "Scorta 9"=FALSE, "Scorta 10"=FALSE}, "AI plc"={"Allarmi 1"=0.0, "Allarmi 2"=0.0, "Stato condensatori"=0.0}}, "Res Ch2"=0.0, "Res Ch2 2"=0.0, "FREDDO res meter"={"Res Ch1"=0.0, "Res Ch2"=0.0, "tAMB"=0.0, "Res Ch3"=0.0}, "Resistenze Res Meter"={"Res Ch1"=0.0, "Res Ch2"=0.0, "Res Ch3"=0.0}, "READ SINUS PENTA"={"Menù Misure motore (M000-M030)"={"Rif vel a regime (int)"=0, "Rif vel a regime (dec)"=0, "Rif vel dopo rampe (int)"=0, "Rif vel dopo rampe (dec)"=0, "RPM motore (int)"=0, "RPM motore (dec)"=0, "FREQout inverter"=0, "Rif coppia a regime(Nm)"=0, "Richiesta di coppia (Nm)"=0, "Coppia generata dal motore(Nm)"=0, "Rif coppia a regime(%)"=0, "Richiesta di coppia (%)"=0, "Coppia generata dal motore(%)"=0, "Coppia max richiesta prima delle rampe(Nm)"=0, "Coppia max richiesta dopo le rampe(Nm)"=0, "Limite di velocità prima delle rampe"=0, "Limite di velocità dopo le rampe"=0, "Coppia max richiesta prima delle rampe(%)"=0, "Coppia max richiesta dopo le rampe(%)"=0, "Rif di flusso"=0, "Corrente di uscita"=0, "Capacità termica del motore"=0, "Tensione di uscita"=0, "Potenza di uscita"=0, "Energia consumata (LSword)"=0, "Energia consumata (MSword)"=0, "Tensione bus DC"=0, "Tensione di rete"=0}, "Menù regolatore PID (M018-M024)"={"Rif PID a regime(%)"=0, "Rif pid dopo rampe(%)"=0, "Retroazione del pid(%)"=0, "Errore del pid(%)"=0, "uscita del pid(%)"=0, "Rif del pid dopo le rampe"=0, "Retroazione del pid"=0}, "Menù ingressi digitali (M031-M036)"={"Ingressi digitali ritardati"=0, "Ingressi digitali istantanei"=0, "Moresettiera comando loc"=0, "Morsett comando da seriale"=0, "Morsett comando bus di campo"=0, "Ing dig ausiliari da morsettiera"=0, "Ing dig ausiliari da seriale"=0}, "Menù riferimenti (M037-M051)"={"Rif analog est REF"=0, "Rif analog est AIN1"=0, "Rif analog est AIN2"=0, "Rif analog est XAIN4"=0, "Rif analog est XAIN5"=0, "Rif velocità da seriale(int)"=0, "Rif velocità bus di campo(int)"=0, "Rif coppia da seriale"=0, "Rif coppia bus di campo"=0, "Rif del PID da seriale"=0, "Rif del PID da bus di campo"=0, "Retroazione del PID da seriale"=0, "Retroazione del PIDda bus di campo"=0, "Rif da encoder"=0, "Rif in frequenza"=0, "Rif velocità da seriale(dec)"=0, "Rif velocità bus di campo(dec)"=0}, "Menù rampe (P009-P033)"={"Tempo di dec rampa di vel 1"=0, "Tempo di acc rampa di vel 2"=0, "Tempo di dec rampa di vel 2"=0, "Tempo di acc rampa di vel 1"=0, "Unità di mis tempi rampe vel 1/2"=0, "Tempo di acc rampa di vel 3"=0, "Tempo di dec rampa di vel 3"=0, "Tempo di acc rampa di vel 4"=0, "Tempo di dec rampa di vel 4"=0, "Unità di mis tempi rampe vel 3/4"=0, "Selettore arrottondam rampe"=0, "Tempo di arrotond iniz rampa acc"=0, "Tempo di arrotond finale rampa acc"=0, "Tempo di arrotond iniz rampa dec"=0, "Tempo di rampa di salita rif coppia"=0, "Tempo di rampa di discesa rif coppia"=0, "Unità di misura rampa coppia"=0, "Tempo rampa acc marcia jog"=0, "Tempo rampa dec marcia jog"=0, "Reset acc ai cambi pendenza"=0, "rampa di acc in fire mode"=0, "rampa di dec in fire mode"=0, "Tempo di arrotond finale rampa dec"=0}, "Menù controllo motore(C008-C128)"={"Numero motori configurati"=0, "Tipo algoritmo di controllo Mot1"=0, "Tipo rif Mot1"=0, "Tensione nominale rete"=0, "Retroaz di vel da encoder Mot1"=0, "Tipo curva V/f Mot1"=0, "Rotazione delle fasi Mot1"=0, "Freq nominale del motore Mot1"=0, "RPM nominali del motore Mot1"=0, "Potenza nominale del motore Mot1"=0, "Corrente nominale del motore Mot1"=0, "Tensione nominale del motore mot1"=0, "Potenza a vuoto del motore Mot1"=0, "Corrente a vuoto del motore Mot1"=0, "Resistenza statorica del motore Mot1"=0, "Induttanza di dispersione Mot1"=0}, "Menù configurazione PID"={"Selezione riferimento n.1"=0, "Selezione retroazione n.1"=0, "Modalità di fuzionamento PID"=0, "Termine derivativo calcolato su err o mis"=0, "Proporz moltiplica deriv e integrale"=0, "Azione del PID"=0}, "ID"=0.0, "Menù uscite digitali"={"MDO4 Inverter pronto"=0}, "Fcarrier"={"Fcarrier Min (Hz)"=0, "Fcarrier Max (Hz)"=0}, "stato inverter M089"=0.0, "Riferimenti"={"Rif tensione"=0, "Rif velocità"=0}}}}}, Variant=w71) -> (data=w55:T20)  [unwired: 1 in, 1 out]
        n19 = feedback #1(FALSE ("Controllo\nPressione")) -> (w68:bool)
        n20 = Unbundle By Name(w55) -> ("CLUSTER PROCESSI.Controllo\nPressione"=w69:bool)
        "Controllo Pressione" <- w69
        n21 = feedback-in #1(w69) -> ()
        n22 = feedback #2() -> (w60:u32)  [unwired: 1 in]
        n23 = case shown="True" w69 {
          selector: w69 -> [_ w156]
          tunnel: w55 -> [w92 _]
          tunnel: w70 -> [w88 w157]
          tunnel: w68 -> [_ w155]
          tunnel: [w86 _] -> w66
          tunnel: [w74 _] -> w65
          tunnel: [w84 _] -> w64
          tunnel: [w83 u32 0] -> w61
          tunnel: w60 -> [w82 _]
          tunnel: [w81 w152] -> w59
          tunnel: T1 {"BooleanV 1"=FALSE, "BooleanV 2"=FALSE, "BooleanV 3"=FALSE, "BooleanV 4"=FALSE, "BooleanV 5"=FALSE, "BooleanV 6"=FALSE, "CTRL BV 2"={"ON"=FALSE, "OFF"=FALSE}, "CTRL BV 3"={"ON"=FALSE, "OFF"=FALSE}, "CTRL BV 4"={"ON"=FALSE, "OFF"=FALSE}, "CTRL BV 5"={"ON"=FALSE, "OFF"=FALSE}, "CTRL BV 6"={"ON"=FALSE, "OFF"=FALSE}, "MTR 1"=FALSE, "DN40%"=0.0, "DN100%"=0.0, "DN250%"=0.0, "DN32"=18.54, "DN100"=2.19, "DN250"=1.87, "MTR 2"=FALSE, "BooleanV 7"=FALSE, "BooleanV 8"=FALSE, "DN25%"=0.0, "DN250_c"=2.24, "CTRL BV 7"={"ON"=FALSE, "OFF"=FALSE}, "CTRL BV 8"={"ON"=FALSE, "OFF"=FALSE}, "DN300%"=0.0, "H 2 [bar]"=1.146, "H 1 [bar]"=0.287, "Rpm\nTorsiometro"=49.82, "Coppia\nTorsiometro"=32.7, "Sonda Velocità"=3000.438, "T 2 [°C]"=18.745, "T 1 [°C]"=7.673, "P [bar]"=9.959, "Livello [m]"=4.374, "MTR 3"=FALSE, "SEL DN40"=FALSE, "SEL DN100"=FALSE, "SEL DN250"=FALSE, "SEL DN300"=FALSE, "SEL DN25"=FALSE} ("SINOTTICO NM") -> [w80 w151]
          frame True {
            w73 = 0  # index pressione misurata
            n24 = Unbundle By Name(w92) -> ("Cluster MISURE.MISURE ALL.INTERFACCIA.AI.Pressioni"=w85:T11[], "CLUSTER PROCESSI.Pressione\nassoluta [bar]"=w86:dbl)
            n25 = local read "Setup pressione"() -> (w79:dbl[])
            n26 = Index Array(array=w79) -> (element #1=w78:dbl, element #2=w77:dbl, element #3=w76:dbl)  [unwired: 3 in]
            n27 = Index Array(array=w85, index=w73) -> (element=w75:T11)
            n28 = Unbundle By Name(w75) -> ("Misura"=w74:dbl)
            n29 = call "CONTROLLO SOGLIE PRESSIONE.vi"("Soglia minima\nassoluta"=w76, "Soglia %"=w78, "Set pressione"=w86, "Pressione misurata"=w74) -> ("UP CONTROL"=w89:bool, "DOWN CONTROL"=w90:bool)  [unwired: 5 in, 1 out]
            n30 = call "CONTROLLO SOGLIE PRESSIONE.vi"("Soglia minima\nassoluta"=w76, "Soglia %"=w77, "Set pressione"=w86, "Pressione misurata"=w74) -> ("IN RANGE"=w91:bool)  [unwired: 5 in, 2 out]
            n31 = Build Array(w91, w90, w89) -> (w84:bool[])
            n32 = Boolean Array To Number(Boolean array=w84) -> (number=w87:u32)
            n33 = case shown="4" w87 {
              selector: w87 -> [w94 w99 w116 w134]
              tunnel: w88 -> [w96 w103 w120 w138]
              tunnel: [w94 w99 w116 w134] -> w83
              tunnel: w82 -> [_ w102 w118 w136]
              tunnel: [w95 w100 w117 w135] -> w81
              tunnel: w80 -> [w93 w98 w115 w133]
              frame 0, Default {
                n34 = property class="Clust"(reference=w96) -> ("Value"=w97:variant)  [unwired: 1 in, 2 out]
                n35 = Variant To Data(type=w93, Variant=w97) -> (data=w95:T1)  [unwired: 1 in, 1 out]
              }
              frame 1 {
                n36 = Not Equal?(x=w99, y=w102) -> (x != y?=w101:bool)
                n37 = case shown="True" w101 {
                  tunnel: w103 -> [w107 w113]
                  tunnel: [w105 w112] -> w100
                  tunnel: w98 -> [w104 w111]
                  frame True {
                    w106 = cluster{"ON":bool, "OFF":bool} {"ON"=FALSE, "OFF"=TRUE} ("CTRL BV 2")
                    n38 = property class="Clust"(reference=w107) -> (reference out=w110:refnum<vi>, "Value"=w108:variant)  [unwired: 1 in, 1 out]
                    n39 = Variant To Data(type=w104, Variant=w108) -> (data=w109:T1)  [unwired: 1 in, 1 out]
                    n40 = Bundle By Name(cluster=w109, "CTRL BV 2"=w106, "CTRL BV 3"=w106) -> (w105:T1)
                    n41 = property class="Clust"(reference=w110, "Val(Sgnl)"=w105) -> ()  [unwired: 1 in, 2 out]
                  }
                  frame False {
                    n42 = property class="Clust"(reference=w113) -> ("Value"=w114:variant)  [unwired: 1 in, 2 out]
                    n43 = Variant To Data(type=w111, Variant=w114) -> (data=w112:T1)  [unwired: 1 in, 1 out]
                  }
                }
              }
              frame 4 {
                n44 = Not Equal?(x=w116, y=w118) -> (x != y?=w119:bool)
                n45 = case shown="False" w119 {
                  tunnel: w120 -> [w125 w131]
                  tunnel: [w123 w130] -> w117
                  tunnel: w115 -> [w121 w129]
                  frame True {
                    n46 = property class="Clust"(reference=w125) -> (reference out=w128:refnum<vi>, "Value"=w126:variant)  [unwired: 1 in, 1 out]
                    n47 = Variant To Data(type=w121, Variant=w126) -> (data=w127:T1)  [unwired: 1 in, 1 out]
                    n48 = Bundle By Name(cluster=w127, "CTRL BV 2"=cluster{"ON":bool, "OFF":bool} {"ON"=TRUE, "OFF"=FALSE}, "CTRL BV 3"=cluster{"ON":bool, "OFF":bool} {"ON"=FALSE, "OFF"=TRUE}) -> (w123:T1)
                    n49 = property class="Clust"(reference=w128, "Val(Sgnl)"=w123) -> ()  [unwired: 1 in, 2 out]
                  }
                  frame False {
                    n50 = property class="Clust"(reference=w131) -> ("Value"=w132:variant)  [unwired: 1 in, 2 out]
                    n51 = Variant To Data(type=w129, Variant=w132) -> (data=w130:T1)  [unwired: 1 in, 1 out]
                  }
                }
              }
              frame 2 {
                n52 = Not Equal?(x=w134, y=w136) -> (x != y?=w137:bool)
                n53 = case shown="True" w137 {
                  tunnel: w138 -> [w143 w149]
                  tunnel: [w141 w148] -> w135
                  tunnel: w133 -> [w139 w147]
                  frame True {
                    n54 = property class="Clust"(reference=w143) -> (reference out=w146:refnum<vi>, "Value"=w144:variant)  [unwired: 1 in, 1 out]
                    n55 = Variant To Data(type=w139, Variant=w144) -> (data=w145:T1)  [unwired: 1 in, 1 out]
                    n56 = Bundle By Name(cluster=w145, "CTRL BV 3"=cluster{"ON":bool, "OFF":bool} {"ON"=TRUE, "OFF"=FALSE} ("CTRL BV 2"), "CTRL BV 2"=cluster{"ON":bool, "OFF":bool} {"ON"=FALSE, "OFF"=TRUE}) -> (w141:T1)
                    n57 = property class="Clust"(reference=w146, "Val(Sgnl)"=w141) -> ()  [unwired: 1 in, 2 out]
                  }
                  frame False {
                    n58 = property class="Clust"(reference=w149) -> ("Value"=w150:variant)  [unwired: 1 in, 2 out]
                    n59 = Variant To Data(type=w147, Variant=w150) -> (data=w148:T1)  [unwired: 1 in, 1 out]
                  }
                }
              }
            }
          }
          frame False {
            n60 = Not Equal?(x=w156, y=w155) -> (x != y?=w154:bool)
            n61 = case shown="False" w154 {
              tunnel: w157 -> [w164 w168]
              tunnel: [w159 w166] -> w152
              tunnel: w151 -> [w158 w165]
              frame True {
                w160 = cluster{"ON":bool, "OFF":bool} {"ON"=FALSE, "OFF"=TRUE} ("CTRL BV 2")
                n62 = property class="Clust"(reference=w164) -> (reference out=w163:refnum<vi>, "Value"=w161:variant)  [unwired: 1 in, 1 out]
                n63 = Variant To Data(type=w158, Variant=w161) -> (data=w162:T1)  [unwired: 1 in, 1 out]
                n64 = Bundle By Name(cluster=w162, "CTRL BV 2"=w160, "CTRL BV 3"=w160) -> (w159:T1)
                n65 = property class="Clust"(reference=w163, "Val(Sgnl)"=w159) -> ()  [unwired: 1 in, 2 out]
              }
              frame False {
                n66 = property class="Clust"(reference=w168) -> ("Value"=w167:variant)  [unwired: 1 in, 2 out]
                n67 = Variant To Data(type=w165, Variant=w167) -> (data=w166:T1)  [unwired: 1 in, 1 out]
              }
            }
          }
        }
        "Set Pressione" <- w66
        "Pressione misurata" <- w65
        "Stato Soglie" <- w64
        n68 = Unbundle By Name(w59) -> ("CTRL BV 2"=→"CTRL BV 2":cluster{"ON":bool, "OFF":bool}, "CTRL BV 3"=→"CTRL BV 3":cluster{"ON":bool, "OFF":bool})
        n69 = feedback-in #2(w61) -> ()
      }
      frame "AVVIA POMPA IN PROVA" {
      }
      frame "FERMA POMPA IN PROVA" {
        n70 = call "INVIA DO A cDAQ.vi"("Array DO"=cluster{"DO":bool, "index":i32}[] [{"DO"=FALSE, "index"=7}]) -> ()  [unwired: 11 in]
      }
      frame "MISURA RESISTENZA RESISTOMAT" {
      }
      frame "OPEN" {
        n71 = global read "Globals.vi" "MONITOR 1"() -> (w180:u8)
        n72 = call <userlib>:"easy open VI panel.vi"("Monitor(1)"=w180, "VI in"=w181) -> ()  [unwired: 9 in, 1 out]
      }
      frame "STOP" {
      }
    }
    n73 = Or(x=w34, y=w35) -> (x .or. y?=w29:bool)
  }
  "error out" <- w14
  n74 = while {
    stop <- w187 stop-if-true
    # "PROCESSI A EVENTI"
    n75 = event shown="[0] \"Stopped\": Value Change" {
      selector: _ -> [_]
      dyn-events: _ -> [_]
      timeout: _ -> [_]
      tunnel: [w188] -> w187
      event "Stopped": Value Change {
        n76 = event-data() -> ("NewVal"=w188:bool)  [unwired: 1 in]
      }
    }
  }
  n77 = property on="Stopped" class="Bool (strict)"("Val(Sgnl)"=w15) -> (error out=w10:errorcluster)  [unwired: 2 in, 1 out]
  n78 = property class="VI"(reference=w11, error in=w10) -> (reference out=w13:refnum<vi>, error out=w9:errorcluster, "FP.State"=w12:T21)
  n79 = case shown="\"Standard\"" w12 {
    tunnel: w13 -> [_ w190]
    tunnel: w9 -> [_ w189]
    frame "Invalid", Default {
    }
    frame "Standard" {
      n80 = invoke class="VI" method="FP.Close"(reference=w190, error in=w189) -> ()  [unwired: 1 in, 3 out]
    }
  }
